vi "AlliGator Get All Ancillary Window Paths.vi"(8 "Error In":errorcluster) -> (0 "Error Out":errorcluster, 3 "AlliGator Window Paths":path[](array[path]))   [LabVIEW 2021, in "AlliGator GUI.lvlib"]
doc: "Returns the paths of all AlliGator windows (except those not close when quitting).\nThis is used when quitting AlliGator."
uses:
  AlliGator GUI.lvlib
  AlliGator Windows List.ctl
  <userlib>/_OpenG.lib/array/array.llb/Filter 1D Array (U16)__ogtk.vi
  <userlib>/_OpenG.lib/array/array.llb/openg_array.lvlib
panel:
  # "see the AlliGator License on the block diagram (Ctrl+E or Window:Show Block Diagram)"
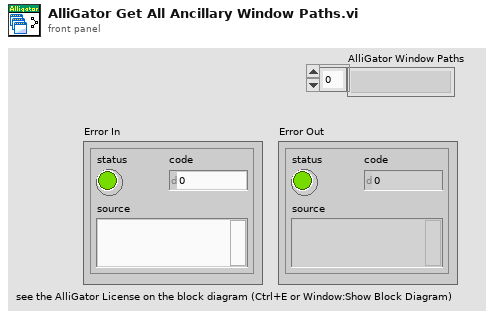
[diagram p1: front panel]
types:
  T1 = typedef "AlliGator GUI.lvlib/AlliGator Windows List.ctl" = enum16{"AlliGator Window", "Settings Window", "Notebook Window", "Dataset Information Window", "Source Image ROI Manager Window", "Phasor Plot ROI Manager Window", "Phasor Harmonic Manager Window", "Histogram Window", "Image Profile Window", "Local Decay Window", "About Window", "Batch Conversion Window", "Shot Noise Influence on Average Lifetime", "Fit Method Benchmark", "AlliGator Alias Definition"}
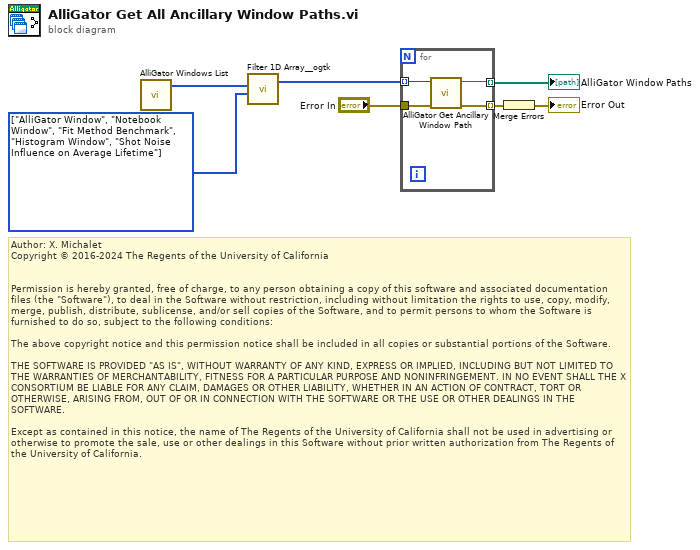
[diagram p0: block diagram]
diagram:
  w2 = T1[] [enum."AlliGator Window", enum."Notebook Window", enum."Fit Method Benchmark", enum."Histogram Window", enum."Shot Noise Influence on Average Lifetime"] items=["AlliGator Window", "Settings Window", "Notebook Window", "Dataset Information Window", "Source Image ROI Manager Window", "Phasor Plot ROI Manager Window", "Phasor Harmonic Manager Window", "Histogram Window", "Image Profile Window", "Local Decay Window", "About Window", "Batch Conversion Window", "Shot Noise Influence on Average Lifetime", "Fit Method Benchmark", "AlliGator Alias Definition"] ("AlliGator Windows List")
  # "Author: X. Michalet\nCopyright © 2016-2024 The Regents of the University of California\n \n\nPermission is hereby granted, free of charge, to any person obtaining a copy of this software and associated documentation files (the \"Software\"), to deal in the Software without restriction, including without limitation the rights to use, copy, modify, merge, publish, distribute, sublicense, and/or sell copies of the Software, and to permit persons to whom the Software is furnished to do so, subject to the following conditions:\n\nThe above copyright notice and this permission notice shall be included in all copies or substantial portions of the Software.\n\nTHE SOFTWARE IS PROVIDED \"AS IS\", WITHOUT WARRANTY OF ANY KIND, EXPRESS OR IMPLIED, INCLUDING BUT NOT LIMITED TO THE WARRANTIES OF MERCHANTABILITY, FITNESS FOR A PARTICULAR PURPOSE AND NONINFRINGEMENT. IN NO EVENT SHALL THE X CONSORTIUM BE LIABLE FOR ANY CLAIM, DAMAGES OR OTHER LIABILITY, WHETHER IN AN ACTION OF CONTRACT, TORT OR OTHERWISE, ARISING FROM, OUT OF OR IN CONNECTION WITH THE SOFTWARE OR THE USE OR OTHER DEALINGS IN THE SOFTWARE.\n\nExcept as contained in this notice, the name of The Regents of the University of California shall not be used in advertising or otherwise to promote the sale, use or other dealings in this Software without prior written authorization from The Regents of the University of California."
  n1 = call "AlliGator Windows List.vi"() -> ("AlliGator Windows List"=w3:T1[])  [unwired: 11 in]
  n2 = call-poly <userlib>:"Filter 1D Array__ogtk.vi"("items to filter"=w2, "array"=w3) -> ("filtered array"=w1:u16[])  [unwired: 4 in, 1 out]
  n3 = for {
    tunnel: w1 -> [w11] mode=indexing
    tunnel: [w10] -> w7 mode=indexing
    tunnel: [w9] -> w6 mode=indexing
    tunnel: "Error In" -> [w8]
    n4 = call "AlliGator Get Ancillary Window Path.vi"("Error In"=w8, "AlliGator Window"=w11) -> ("Error Out"=w9:errorcluster, "VI Path"=w10:path)  [unwired: 8 in]
  }
  "AlliGator Window Paths" <- w7
  n5 = Merge Errors(w6) -> (→"Error Out":errorcluster)
